vi "BuildMeasurementRow.vi"() -> ()   [LabVIEW 2022 SP3]
uses:
  Anemometry Sub Vis/Controls/MeasurementLocation.ctl
  Anemometry Sub Vis/Gen Trav/Spacing.ctl
  Anemometry Sub Vis/Controls/Multi_run_mode.ctl
panel:
  out "Row Out":T3 {"Carrier_2 Q (l/min)" format="%#.2f"; "Row Duration (mins)" format="%#.1f"; "Row No" min=0; "Trace Gas Concentration (%)" min=0.0 format="%#_4f"; "Carrier_1 Q (l/min)" format="%#.2f"; "Tunnel Speed" format="%#.2f"; "Start X" format="%#.2f"; "Start Y" format="%#.2f"; "Start Z" format="%#.2f"; "End X" format="%#.2f"; "End Y" format="%#.2f"; "End Z" format="%#.2f"; "Averaging time (min)" min=0.0 format="%#.2f"}
  in  "Location":T4 caption="X                          Y                    RoofZ                        Name"
  in  "ZsAboveRoof":sgl[](array[numeric])=[16.8, 25.4, 33.9]
  # "X           Y            Z"
  # "Start"
  # "End"
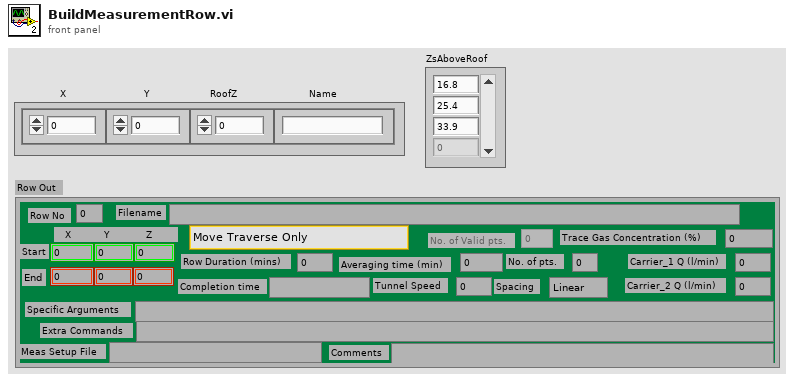
[diagram p1: front panel]
types:
  T1 = typedef "Spacing.ctl" = enum16{"Linear", "Log", "Gauss", "Specified", "N/A"}
  T2 = typedef "Multi_run_mode.ctl" = enum16{"Move Traverse Only", "Set Tunnel Speed Only", "Set Source Only", "Set Measurement Conditions", "Single Measurement", "Vertical Profile", "Lateral Profile", "Longitudinal Profile", "Multi-Axis Profile", "Explore Volume", "Auto Calibrate", "Meas Fast FID Bkgnd", "Check Beam Power", "Scanning Valve Measurement", "Run VI Named:", "Set ADAM Ch", "Wait (minutes)", "Send Message", "Synchronize With:", "Fall Back to this Row", "Turn Off Row Repeating", "Traverse 3D Volume", "Blank Row", "Jump to Fall Back Row"}
  T3 = cluster{"Start X":sgl, "Start Y":sgl, "Start Z":sgl, "End X":sgl, "End Y":sgl, "End Z":sgl, "No. of pts.":i32, "Spacing":T1, "Filename":path, "Tunnel Speed":dbl, "Averaging time (min)":dbl, "Extra Commands":string, "Carrier_1 Q (l/min)":dbl, "Carrier_2 Q (l/min)":dbl, "Trace Gas Concentration (%)":dbl, "Specific Arguments":string, "Comments":string, "Row No":i32, "Row Type Selector":T2, "Completion time":string, "Row Duration (mins)":dbl, "No. of Valid pts.":i32, "Meas Setup File":string}
  T4 = typedef "MeasurementLocation.ctl" = cluster{"X":sgl, "Y":sgl, "LocalZ0":sgl, "Name":string}
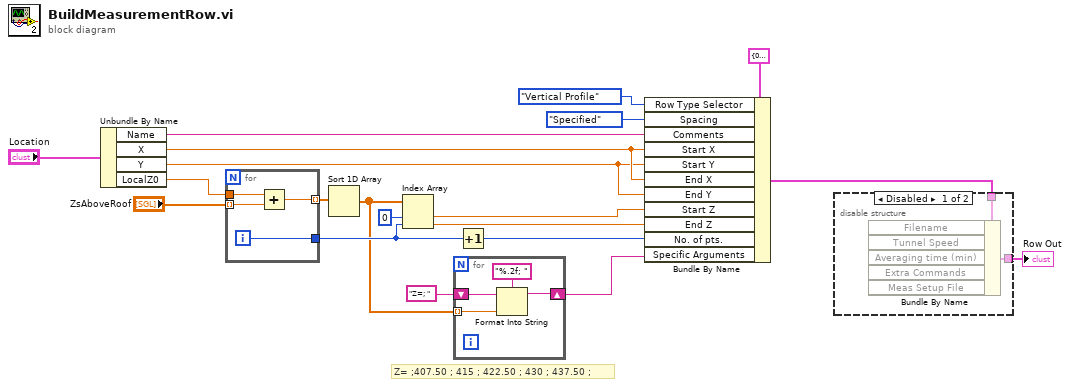
[diagram p0: block diagram]
diagram:
  # "Z= ;407.50 ; 415 ; 422.50 ; 430 ; 437.50 ;"
  n1 = Unbundle By Name("Location") -> ("Name"=w9:string, "X"=w2:sgl, "Y"=w1:sgl, "LocalZ0"=w17:sgl)
  n2 = for {
    tunnel: "ZsAboveRoof" -> [w24] mode=indexing
    tunnel: w17 -> [w23]
    tunnel: [w22] -> w16 mode=indexing
    tunnel: [w21] -> w13
    i -> [w21]
    n3 = Add(x=w23, y=w24) -> (x+y=w22:sgl)
  }
  n4 = Sort 1D Array(array=w16) -> (sorted array=w7:sgl[])
  n5 = Index Array(array=w7, index #1=0 ("index"), index #2=w13) -> (element #1=w3:sgl, element #2=w12:sgl)
  n6 = for {
    tunnel: w7 -> [w27] mode=indexing
    shift-right: [w26] -> w5
    shift-left: "Z=; " -> [w28]
    n7 = Format Into String(format string="%.2f; ", initial string=w28, w27) -> (resulting string=w26:string)  [unwired: 1 in, 1 out]
  }
  n8 = Increment(x=w13) -> (x+1=w15:i32)
  n9 = Bundle By Name(cluster=T3 {"Start X"=0.0, "Start Y"=0.0, "Start Z"=0.0, "End X"=0.0, "End Y"=0.0, "End Z"=0.0, "No. of pts."=0, "Spacing"=enum."Linear", "Filename"=path "", "Tunnel Speed"=0.0, "Averaging time (min)"=0.0, "Extra Commands"="", "Carrier_1 Q (l/min)"=0.0, "Carrier_2 Q (l/min)"=0.0, "Trace Gas Concentration (%)"=0.0, "Specific Arguments"="", "Comments"="", "Row No"=0, "Row Type Selector"=enum."Move Traverse Only", "Completion time"="", "Row Duration (mins)"=0.0, "No. of Valid pts."=0, "Meas Setup File"=""} ("RowTemplate"), "Row Type Selector"=Multi_run_mode."Vertical Profile", "Spacing"=Spacing."Specified", "Comments"=w9, "Start X"=w2, "Start Y"=w1, "End X"=w2, "End Y"=w1, "Start Z"=w3, "End Z"=w12, "No. of pts."=w15, "Specific Arguments"=w5) -> (w8:T3)
  n10 = disable-structure shown="Disabled" {
    disable-tunnel: w8 -> [w30 w31]
    disable-tunnel: [w29 w31] -> w4
    frame Disabled {
      n11 = Bundle By Name(cluster=w30) -> (w29:T3)  [unwired: 5 in]
    }
    frame Enabled {
    }
  }
  "Row Out" <- w4
